vi "Forward Kinematics Demo.vi"() -> ()   [LabVIEW 2017, in "NI_Kinematics.lvlib"]
uses:
  <vilib>/robotics/Kinematics/NI_Kinematics.lvlib
  <vilib>/Analysis/Matrix/Datatypes/RealMatrix.ctl
  <vilib>/robotics/Kinematics/Robot/Forward Kinematics (Trajectory).vi
  <vilib>/robotics/Kinematics/Generate Joint Trajectory (Array).vi
  <vilib>/robotics/Kinematics/Robot/Forward Kinematics (Point).vi
  <vilib>/robotics/Kinematics/Robot/NI_Robotics_Serial Robot Arm.lvclass
  <vilib>/Analysis/Matrix/NI_Matrix.lvlib
panel:
  out "Joint Positions":dbl[][](array[numeric])
  out "end effector transform":T1
  out "Tau":dbl[][][](array[numeric])
  out "Time (ms)":u32
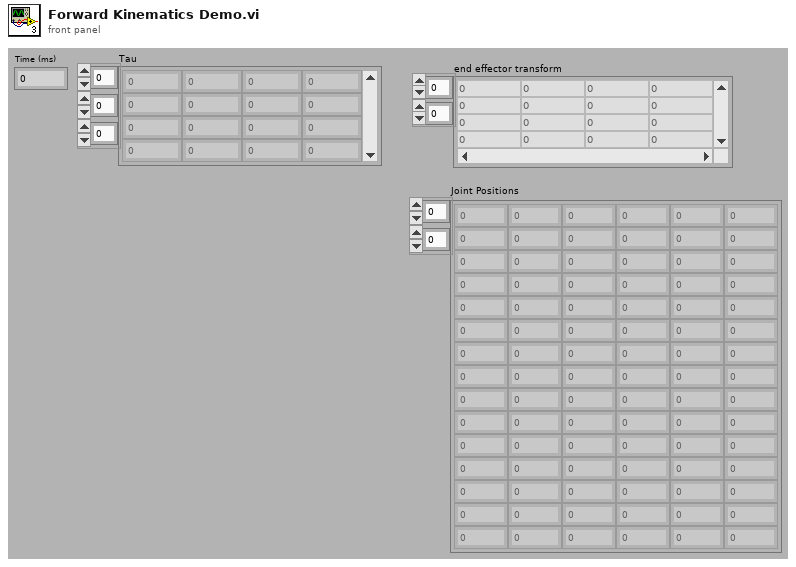
[diagram p1: front panel]
types:
  T1 = typedef "NI_Matrix.lvlib/RealMatrix.ctl" = dbl[][]
  T2 = typedef "NI_Robotics_Serial Robot Arm.lvclass/Robot Pose.ctl" = cluster{"name":string, "description":string, "joint positions":dbl[]}
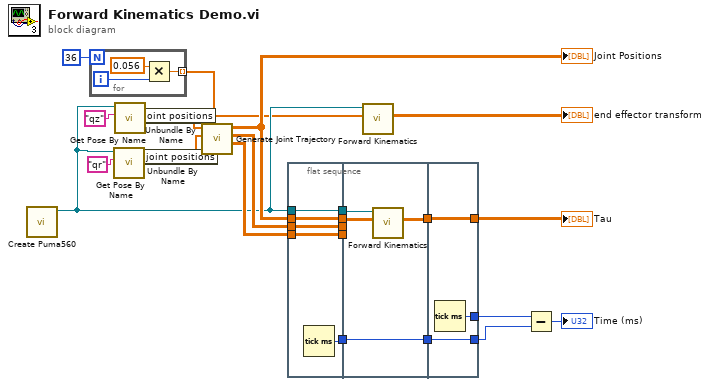
[diagram p0: block diagram]
diagram:
  n1 = call <vilib>:"Create Puma560.vi"() -> ("Puma560 Robot"=w10:refnum<class "NI_Robotics_Serial Robot Arm.lvclass">)  [unwired: 1 in, 10 out]
  n2 = for {
    N: 36 -> [_]
    tunnel: [w25] -> w11 mode=indexing
    i -> [w27]
    n3 = Multiply(x=0.056, y=w27) -> (x*y=w25:dbl)
  }
  n4 = call <vilib>:"Get Pose By Name.vi"("name"="qr" ("Name"), "serial arm in"=w10) -> ("serial arm pose"=w18:T2)  [unwired: 7 in, 2 out]
  n5 = call <vilib>:"Get Pose By Name.vi"("name"="qz" ("Name"), "serial arm in"=w10) -> ("serial arm pose"=w17:T2)  [unwired: 7 in, 2 out]
  n6 = Unbundle By Name(w17) -> ("joint positions"=w9:dbl[])
  n7 = Unbundle By Name(w18) -> ("joint positions"=w16:dbl[])
  n8 = call-poly <vilib>:"Generate Joint Trajectory.vi"("intermediate points"=w11, "end joint positions"=w16, "start joint positions"=w9) -> ("joint acceleration trajectory"=w13:dbl[][], "joint velocity trajectory"=w14:dbl[][], "joint position trajectory"=w15:dbl[][])  [unwired: 5 in, 1 out]
  "Joint Positions" <- w15
  n9 = flat-sequence {
    tunnel: w10 -> [w32]
    tunnel: [w32] -> w7
    tunnel: [w31] -> w6
    tunnel: w15 -> [w30]
    tunnel: w14 -> [w29]
    tunnel: w13 -> [w28]
    tunnel: [w30] -> w5
    tunnel: [w29] -> w4
    tunnel: [w28] -> w3
    tunnel: w7 -> [w33]
    tunnel: w6 -> [w36]
    tunnel: [w36] -> w2
    tunnel: [w34] -> w1
    tunnel: w5 -> [w35]
    tunnel: w4 -> [_]
    tunnel: w3 -> [_]
    tunnel: [w39] -> w23
    tunnel: w2 -> [w39]
    tunnel: [w38] -> w24
    tunnel: w1 -> [w37]
    tunnel: [w37] -> w21
    frame #0 {
      n10 = Tick Count (ms)() -> (millisecond timer value=w31:u32)
    }
    frame #1 {
      n11 = call-poly <vilib>:"Forward Kinematics.vi"("joint position trajectory"=w35, "serial arm in"=w33) -> ("end effector transforms"=w34:dbl[][][])  [unwired: 7 in, 2 out]
    }
    frame #2 {
      n12 = Tick Count (ms)() -> (millisecond timer value=w38:u32)
    }
  }
  n13 = call-poly <vilib>:"Forward Kinematics.vi"("joint positions"=w9, "serial arm in"=w10) -> ("end effector transform"=→"end effector transform":T1)  [unwired: 7 in, 2 out]
  n14 = Subtract(x=w24, y=w23) -> (x-y=→"Time (ms)":u32)
  "Tau" <- w21
